vi "GUI AWG setup.vi"(11 "awg":T3={"AWG type"=enum."Agilent 331xxA to 332xxA", "FGEN Resource Name"="", "Source (Onboard Clock)"="OnboardClock", "FGEN Channel"="0", "awg lib session"={"type"=enum."Agilent 331xxA to 332xxA", "VISA"="", "enable 10MHz ref"=FALSE, "cmi ckd2"={"VISA"="", "clock source"=enum."Auto", "manual ref clk"=FALSE, "ref clock [Hz]"=0.0, "div mode"=enum."Set divisor directly"}, "cmi sync v3"={"VISA"="", "baud rate [bd/s]"=115200, "source"=enum."Auto", "hv range"=enum."1kV", "fsrc is fixed"=FALSE, "fsrc [Hz]"=10000000.0, "freq integ [s]"=1.0, "freq filter"=5, "trig level"=enum."TTL 5V", "chn1 mode"=enum."Source divider", "chn1 level"=enum."Positive 5V", "chn2 mode"=enum."Source divider", "chn2 level"=enum."Positive 5V", "chn2 div"=1, "chn3 mode"=enum."Chn 1 Active", "chn3 level"=enum."Positive 5V", "chn1 div entry"=enum."Calculate nearest divisor from measured fx", "chn1 dev limit [%]"=1.0, "chn1 check dev"=FALSE}, "trigger"={"source"=enum."Immediate", "level [V]"=0.0, "coupling"=enum."DC", "slope"=enum."POS"}, "HMF2500 cfg"={"Baud Rate"=9600, "Parity"=0, "Data Bits"=8, "Flow Control"=4}}} {"awg lib session"."HMF2500 cfg"."Flow Control" items=["None", "XON/XOFF", "RTS/CTS", "XON/XOFF & RTS/CTS", "DTR/DSR", "XON/XOFF & DTR/DSR"]; "awg lib session"."HMF2500 cfg"."Data Bits" items=["7"=7, "8"=8]; "awg lib session"."HMF2500 cfg"."Parity" items=["None", "Odd", "Even", "Mark", "Space"]; "awg lib session"."HMF2500 cfg"."Baud Rate" items=["300"=300, "600"=600, "1200"=1200, "2400"=2400, "4800"=4800, "9600"=9600, "19200"=19200]; "awg lib session"."cmi sync v3"."chn2 div" min=1 max=100000000 step=1; "awg lib session"."cmi sync v3"."fsrc [Hz]" format="%_8p"}) -> (3 "awg out":T3={"AWG type"=enum."Agilent 331xxA to 332xxA", "FGEN Resource Name"="", "Source (Onboard Clock)"="OnboardClock", "FGEN Channel"="0", "awg lib session"={"type"=enum."Agilent 331xxA to 332xxA", "VISA"="", "enable 10MHz ref"=FALSE, "cmi ckd2"={"VISA"="", "clock source"=enum."Auto", "manual ref clk"=FALSE, "ref clock [Hz]"=0.0, "div mode"=enum."Set divisor directly"}, "cmi sync v3"={"VISA"="", "baud rate [bd/s]"=115200, "source"=enum."Auto", "hv range"=enum."1kV", "fsrc is fixed"=FALSE, "fsrc [Hz]"=10000000.0, "freq integ [s]"=1.0, "freq filter"=5, "trig level"=enum."TTL 5V", "chn1 mode"=enum."Source divider", "chn1 level"=enum."Positive 5V", "chn2 mode"=enum."Source divider", "chn2 level"=enum."Positive 5V", "chn2 div"=1, "chn3 mode"=enum."Chn 1 Active", "chn3 level"=enum."Positive 5V", "chn1 div entry"=enum."Calculate nearest divisor from measured fx", "chn1 dev limit [%]"=1.0, "chn1 check dev"=FALSE}, "trigger"={"source"=enum."Immediate", "level [V]"=0.0, "coupling"=enum."DC", "slope"=enum."POS"}, "HMF2500 cfg"={"Baud Rate"=9600, "Parity"=0, "Data Bits"=8, "Flow Control"=4}}} {"awg lib session"."HMF2500 cfg"."Flow Control" items=["None", "XON/XOFF", "RTS/CTS", "XON/XOFF & RTS/CTS", "DTR/DSR", "XON/XOFF & DTR/DSR"]; "awg lib session"."HMF2500 cfg"."Data Bits" items=["7"=7, "8"=8]; "awg lib session"."HMF2500 cfg"."Parity" items=["None", "Odd", "Even", "Mark", "Space"]; "awg lib session"."HMF2500 cfg"."Baud Rate" items=["300"=300, "600"=600, "1200"=1200, "2400"=2400, "4800"=4800, "9600"=9600, "19200"=19200]; "awg lib session"."cmi sync v3"."chn2 div" min=1 max=100000000 step=1; "awg lib session"."cmi sync v3"."fsrc [Hz]" format="%_8p"})   [LabVIEW 2020]
doc: "Use this template to build a producer/consumer design pattern with events to produce queue items. Use this design pattern instead of the User Interface Event Handler pattern for user interfaces when you want to execute code asynchronously in response to an event without slowing the user interface responsiveness."
uses:
  General AWG/Type definitions/AWG.ctl
  General AWG/Type definitions/AWG type.ctl
  <instrlib>/niFgen/niFgen.llb/niFgen_ctl Sample Clock Source Values (Ring).ctl
  external libraries/AWG/AWG Session.ctl
  external libraries/AWG/AWG Type.ctl
  external libraries/AWG/CMI Clock Divider v2/CMI ckd2 Session.ctl
  external libraries/AWG/CMI Clock Divider v2/CMI ckd2 Source Mode.ctl
  external libraries/AWG/CMI Clock Divider v2/CMI ckd2 Divisor Mode.ctl
  external libraries/AWG/CMI Sync V3/CMI Sync V3 session.ctl
  external libraries/AWG/CMI Sync V3/Configure/CMI Sync V3 Reference Clock Source.ctl
  external libraries/AWG/CMI Sync V3/Configure/CMI Sync V3 HV input Range.ctl
  external libraries/AWG/CMI Sync V3/Configure/CMI Sync V3 Trigger Input Level.ctl
  external libraries/AWG/CMI Sync V3/Configure/CMI Sync V3 Channel 1 Mode.ctl
  external libraries/AWG/CMI Sync V3/Configure/CMI Sync V3 Channel Output Levels.ctl
  external libraries/AWG/CMI Sync V3/Configure/CMI Sync V3 Channel 2 Mode.ctl
  external libraries/AWG/CMI Sync V3/Configure/CMI Sync V3 Channel 3 Mode.ctl
  external libraries/AWG/CMI Sync V3/Configure/CMI Sync V3 Channel 1 Divisor Entry Mode.ctl
  external libraries/externals needed for AWG/ADC Trig Config.ctl
  external libraries/externals needed for AWG/ADC Trig Mode Source.ctl
  external libraries/externals needed for AWG/ADC Trig Coupling.ctl
  external libraries/externals needed for AWG/ADC Trig Slope.ctl
  external libraries/AWG/RaS HMF2500/HMF2500 Config.ctl
  <vilib>/Utility/error.llb/DialogType.ctl
  <vilib>/Utility/error.llb/Error Cluster From Error Code.vi
  <vilib>/ErrorRing/Error Ring.xnode
  external libraries/varilib/varilib.lvlib
  external libraries/AWG/AWG.lvlib
  external libraries/AWG/CMI Sync V3/CMI Sync Unit V3.lvlib
panel:
  in  "AWG type":T1
  in  "Channel":string
  in  "Clock Source":T2="OnboardClock"
  in  "FGEN Resource Name":refnum<k15>
  in  "Enable 10MHz ref":bool
  in  "VISA":refnum<visa-resource-name>
  in  "control panel":bool
  out "gui_elements":refnum<vi>[](array[refnum])
  out "Status":string
  in  "save_and_quit":bool
  in  "test":bool
  in  "cancel":bool
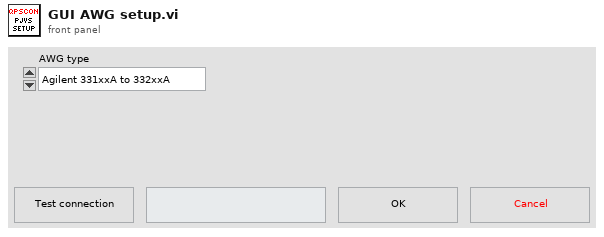
[diagram p1: front panel]
types:
  T1 = typedef "AWG type.ctl" = enum16{"Agilent 331xxA to 332xxA", "Agilent 335xxA to 336xxA", "Tektronix AFG3101C", "R&S HMF25xx", "CMI Clock Divider v2", "CMI Sync Unit V3", "FGEN NI 5413", "Supracon PJVS Generator", "dummy"}
  T2 = typedef "niFgen_ctl Sample Clock Source Values (Ring).ctl" = string
  T3 = typedef "AWG.ctl" = cluster{"AWG type":T1, "FGEN Resource Name":refnum<k15>, "Source (Onboard Clock)":T2, "FGEN Channel":string, "awg lib session":T4}
  T4 = typedef "AWG.lvlib/AWG Session.ctl" = cluster{"type":T5, "VISA":refnum<visa-resource-name>, "enable 10MHz ref":bool, "cmi ckd2":T6, "cmi sync v3":T9, "trigger":T18, "HMF2500 cfg":T22}
  T5 = typedef "AWG.lvlib/AWG Type.ctl" = enum16{"Agilent 331xxA to 332xxA", "Agilent 335xxA to 336xxA", "Tektronix AFG3101C", "R&S HMF25xx", "CMI Clock Divider v2", "CMI Sync Unit V3", "dummy"}
  T6 = typedef "AWG.lvlib/CMI ckd2 Session.ctl" = cluster{"VISA":refnum<visa-resource-name>, "clock source":T7, "manual ref clk":bool, "ref clock [Hz]":dbl, "div mode":T8}
  T7 = typedef "AWG.lvlib/CMI ckd2 Source Mode.ctl" = enum16{"Auto", "LF clock", "HF clock", "Internal"}
  T8 = typedef "AWG.lvlib/CMI ckd2 Divisor Mode.ctl" = enum16{"Set divisor directly", "Set divisor by frequency"}
  T9 = typedef "AWG.lvlib/CMI Sync Unit V3.lvlib/CMI Sync V3 session.ctl" = cluster{"VISA":refnum<visa-resource-name>, "baud rate [bd/s]":i32, "source":T10, "hv range":T11, "fsrc is fixed":bool, "fsrc [Hz]":dbl, "freq integ [s]":dbl, "freq filter":i32, "trig level":T12, "chn1 mode":T13, "chn1 level":T14, "chn2 mode":T15, "chn2 level":T14, "chn2 div":i32, "chn3 mode":T16, "chn3 level":T14, "chn1 div entry":T17, "chn1 dev limit [%]":dbl, "chn1 check dev":bool}
  T10 = typedef "AWG.lvlib/CMI Sync Unit V3.lvlib/CMI Sync V3 Reference Clock Source.ctl" = enum16{"Auto", "Internal", "Logic", "Sine", "HV"}
  T11 = typedef "AWG.lvlib/CMI Sync Unit V3.lvlib/CMI Sync V3 HV input Range.ctl" = enum16{"10V", "60V", "250V", "1kV"}
  T12 = typedef "AWG.lvlib/CMI Sync Unit V3.lvlib/CMI Sync V3 Trigger Input Level.ctl" = enum16{"LVCMOS 3V3", "TTL 5V"}
  T13 = typedef "AWG.lvlib/CMI Sync Unit V3.lvlib/CMI Sync V3 Channel 1 Mode.ctl" = enum16{"Source divider", "DDS absolute", "DDS ratio", "DDS ratio M/N"}
  T14 = typedef "AWG.lvlib/CMI Sync Unit V3.lvlib/CMI Sync V3 Channel Output Levels.ctl" = enum16{"Positive 3V3", "Negative 3V3", "Positive 5V", "Negative 5V"}
  T15 = typedef "AWG.lvlib/CMI Sync Unit V3.lvlib/CMI Sync V3 Channel 2 Mode.ctl" = enum16{"Source divider", "Chn 1 divide"}
  T16 = typedef "AWG.lvlib/CMI Sync Unit V3.lvlib/CMI Sync V3 Channel 3 Mode.ctl" = enum16{"Chn 1 Active", "Chn 2 Active", "Chn 1 Trigger", "Chn 2 Trigger", "Gate", "PPS", "10MHz"}
  T17 = typedef "AWG.lvlib/CMI Sync Unit V3.lvlib/CMI Sync V3 Channel 1 Divisor Entry Mode.ctl" = enum16{"Set divisor directly", "Calculate nearest divisor from measured fx"}
  T18 = typedef "ADC Trig Config.ctl" = cluster{"source":T19, "level [V]":dbl, "coupling":T20, "slope":T21}
  T19 = typedef "ADC Trig Mode Source.ctl" = enum16{"Immediate", "External", "Level"}
  T20 = typedef "ADC Trig Coupling.ctl" = enum16{"DC", "AC"}
  T21 = typedef "ADC Trig Slope.ctl" = enum16{"POS", "NEG"}
  T22 = typedef "AWG.lvlib/HMF2500 Config.ctl" = cluster{"Baud Rate":u32, "Parity":u16, "Data Bits":u16, "Flow Control":u16}
  T23 = typedef "DialogType.ctl" = u16
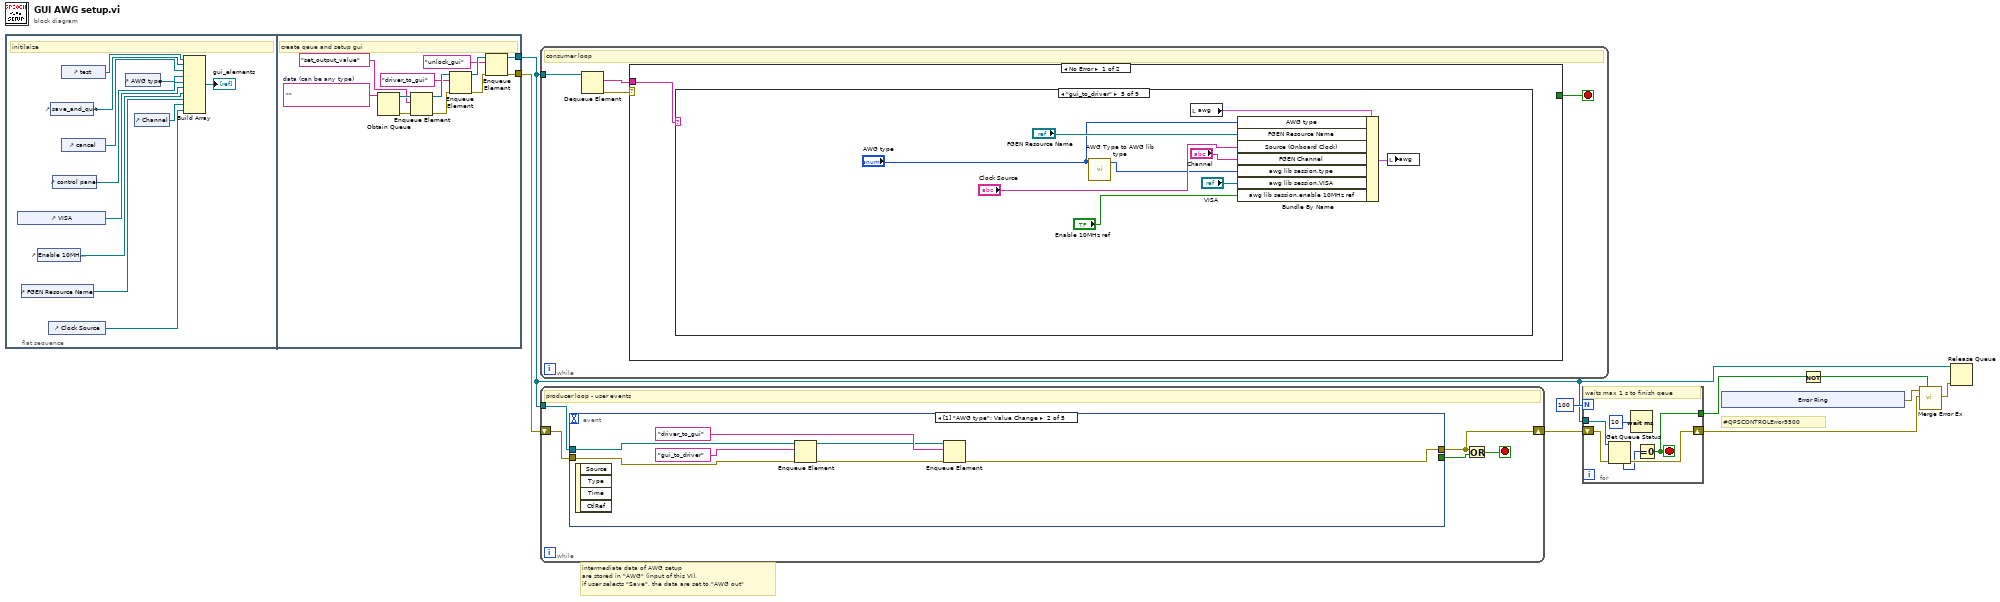
[diagram p0: block diagram]
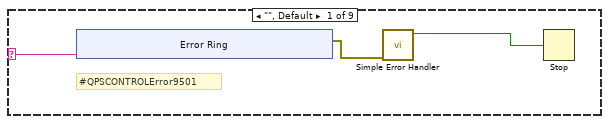
[diagram p2: hidden frame]
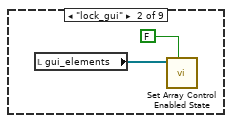
[diagram p3: hidden frame]
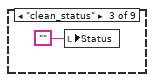
[diagram p4: hidden frame]
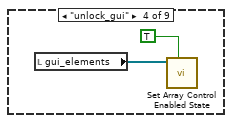
[diagram p5: hidden frame]
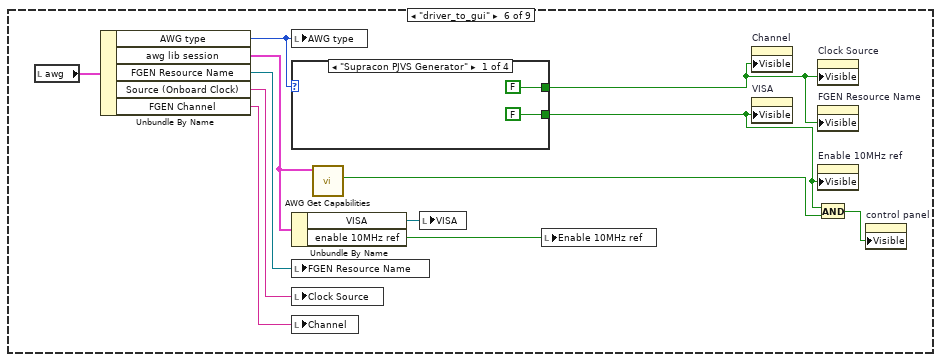
[diagram p6: hidden frame]
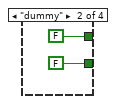
[diagram p7: hidden frame]
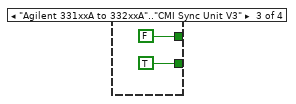
[diagram p8: hidden frame]
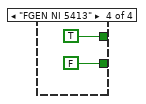
[diagram p9: hidden frame]
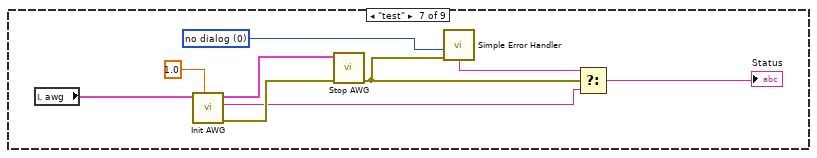
[diagram p10: hidden frame]
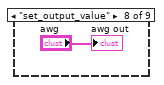
[diagram p11: hidden frame]
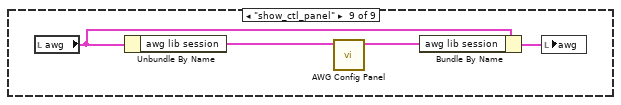
[diagram p12: hidden frame]
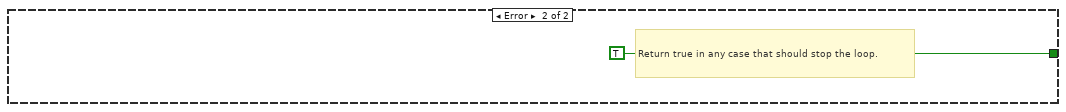
[diagram p13: hidden frame]
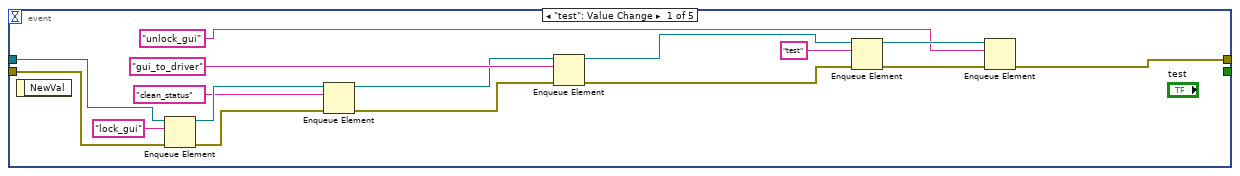
[diagram p14: hidden frame]
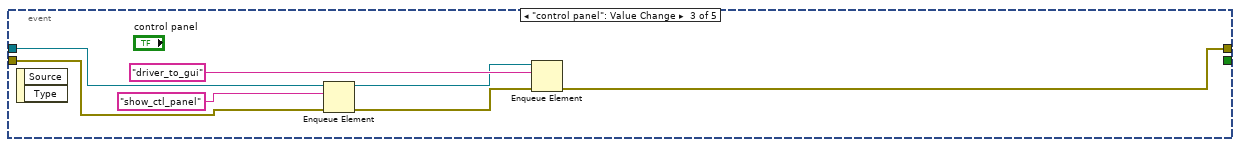
[diagram p15: hidden frame]
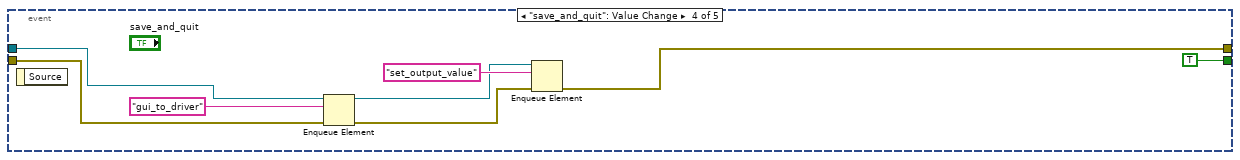
[diagram p16: hidden frame]
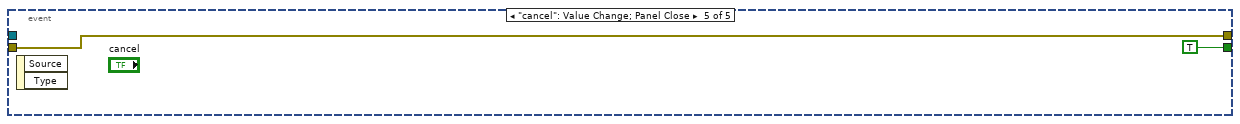
[diagram p17: hidden frame]
diagram:
  # "#QPSCONTROLError9500"
  # "intermediate data of AWG setup\nare stored in \"AWG\" (input of this VI),\nif user selects \"Save\", the data are set to \"AWG out\""
  n1 = flat-sequence {
    tunnel: [w23] -> w2
    tunnel: [w21] -> w1
    frame #0 {
      # "initilaize"
      n2 = control-ref of="VISA"() -> (w15:refnum<vi>)
      n3 = control-ref of="FGEN Resource Name"() -> (w13:refnum<vi>)
      n4 = control-ref of="Enable 10MHz ref"() -> (w14:refnum<vi>)
      n5 = control-ref of="Clock Source"() -> (w11:refnum<vi>)
      n6 = control-ref of="save_and_quit"() -> (w19:refnum<vi>)
      n7 = control-ref of="control panel"() -> (w16:refnum<vi>)
      n8 = control-ref of="test"() -> (w20:refnum<vi>)
      n9 = control-ref of="cancel"() -> (w18:refnum<vi>)
      n10 = control-ref of="AWG type"() -> (w10:refnum<vi>)
      n11 = control-ref of="Channel"() -> (w12:refnum<vi>)
      n12 = Build Array(w20, w19, w18, w10, w16, w15, w14, w13, w12, w11) -> (→"gui_elements":refnum<vi>[])
    }
    frame #1 {
      w22 = ""  # data (can be any type)
      # "create qeue and setup gui"
      n13 = Obtain Queue(element data type=w22) -> (queue out=w27:refnum<queue>, error out=w29:errorcluster)  [unwired: 4 in, 1 out]
      n14 = Enqueue Element(queue=w27, element="set_output_value", error in (no error)=w29) -> (queue out=w28:refnum<queue>, error out=w30:errorcluster)  [unwired: 1 in, 1 out]
      n15 = Enqueue Element(queue=w28, element="driver_to_gui", error in (no error)=w30) -> (queue out=w32:refnum<queue>, error out=w31:errorcluster)  [unwired: 1 in, 1 out]
      n16 = Enqueue Element(queue=w32, element="unlock_gui", error in (no error)=w31) -> (queue out=w23:refnum<queue>, error out=w21:errorcluster)  [unwired: 1 in, 1 out]
    }
  }
  n17 = while {
    tunnel: w2 -> [w36]
    stop <- w33 stop-if-true
    # "consumer loop"
    n18 = Dequeue Element(queue=w36) -> (element=w34:string, error out=w35:errorcluster)  [unwired: 2 in, 2 out]
    n19 = case shown="No Error" w35 {
      tunnel: w34 -> [w37 _]
      tunnel: [_ TRUE] -> w33
      frame No Error {
        n20 = case shown="\"gui_to_driver\"" w37 {
          selector: w37 -> [w38 _ _ _ _ _ _ _ _]
          frame "", Default {
            # "#QPSCONTROLError9501"
            n21 = xnode "Error Ring"("parameter 0"=w38) -> ("error out"=w40:errorcluster)
            n22 = call <vilib>:"Simple Error Handler.vi"("error in (no error)"=w40) -> ("error?"=w39:bool)  [unwired: 4 in, 4 out]
            n23 = Stop(stop? (T)=w39) -> ()
          }
          frame "lock_gui" {
            n24 = local read "gui_elements"() -> (w49:refnum<vi>[])
            n25 = call "Set Array Control Enabled State.vi"("enabled (T)"=FALSE, "reference array in"=w49) -> ()  [unwired: 8 in, 2 out]
          }
          frame "clean_status" {
            n26 = local write "Status"("") -> ()
          }
          frame "unlock_gui" {
            n27 = local read "gui_elements"() -> (w52:refnum<vi>[])
            n28 = call "Set Array Control Enabled State.vi"("enabled (T)"=TRUE, "reference array in"=w52) -> ()  [unwired: 8 in, 2 out]
          }
          frame "gui_to_driver" {
            n29 = call "AWG Type to AWG lib type.vi"("AWG type"="AWG type") -> ("AWG lib type"=w54:T5)  [unwired: 10 in]
            n30 = local read "awg"() -> (w60:T3)
            n31 = Bundle By Name(cluster=w60, "AWG type"="AWG type", "FGEN Resource Name"="FGEN Resource Name", "Source (Onboard Clock)"="Clock Source", "FGEN Channel"="Channel", "awg lib session.type"=w54, "awg lib session.VISA"="VISA", "awg lib session.enable 10MHz ref"="Enable 10MHz ref") -> (w61:T3)
            n32 = local write "awg"(w61) -> ()
          }
          frame "driver_to_gui" {
            n33 = local read "awg"() -> (w71:T3)
            n34 = Unbundle By Name(w71) -> ("AWG type"=w62:T1, "awg lib session"=w63:T4, "FGEN Resource Name"=w64:refnum<k15>, "Source (Onboard Clock)"=w65:T2, "FGEN Channel"=w66:string)
            n35 = local write "AWG type"(w62) -> ()
            n36 = case shown="\"Supracon PJVS Generator\"" w62 {
              tunnel: [FALSE ("x") FALSE ("x") TRUE ("x") FALSE ("x")] -> w68
              tunnel: [FALSE ("Visible") FALSE ("Visible") FALSE ("Visible") TRUE ("Visible")] -> w67
              frame "Supracon PJVS Generator" {
              }
              frame "dummy" {
              }
              frame "Agilent 331xxA to 332xxA".."CMI Sync Unit V3" {
              }
              frame "FGEN NI 5413" {
              }
            }
            n37 = Unbundle By Name(w63) -> ("VISA"=w72:refnum<visa-resource-name>, "enable 10MHz ref"=w73:bool)
            n38 = local write "FGEN Resource Name"(w64) -> ()
            n39 = local write "Clock Source"(w65) -> ()
            n40 = local write "Channel"(w66) -> ()
            n41 = call "AWG Get Capabilities.vi"("awg session"=w63) -> ("has cfg panel?"=w70:bool)  [unwired: 6 in, 4 out]
            n42 = local write "VISA"(w72) -> ()
            n43 = local write "Enable 10MHz ref"(w73) -> ()
            n44 = property on="Channel" class="Str"("Visible"=w67) -> ()  [unwired: 2 in, 2 out]
            n45 = property on="VISA" class="VISAName"("Visible"=w68) -> ()  [unwired: 2 in, 2 out]
            n46 = property on="Clock Source" class="CmbBox (strict)"("Visible"=w67) -> ()  [unwired: 2 in, 2 out]
            n47 = property on="FGEN Resource Name" class="IVIName"("Visible"=w67) -> ()  [unwired: 2 in, 2 out]
            n48 = property on="Enable 10MHz ref" class="Bool (strict)"("Visible"=w68) -> ()  [unwired: 2 in, 2 out]
            n49 = And(x=w68, y=w70) -> (x .and. y?=w69:bool)
            n50 = property on="control panel" class="Bool"("Visible"=w69) -> ()  [unwired: 2 in, 2 out]
          }
          frame "test" {
            w90 = T23 0 items=["no dialog", "OK message", "continue or stop message", "OK message + warnings", "continue/stop + warnings"] ("type of dialog (OK msg:1)")
            n51 = local read "awg"() -> (w87:T3)
            n52 = call "Init AWG.vi"("Trigger frequency  (Hz)"=1.0, "AWG"=w87) -> ("error out"=w84:errorcluster, "Init status"=w83:string, "AWG out"=w86:T3)  [unwired: 7 in]
            n53 = call "Stop AWG.vi"("error in (no error)"=w84, "AWG"=w86) -> ("error out"=w82:errorcluster)  [unwired: 8 in, 1 out]
            n54 = call <vilib>:"Simple Error Handler.vi"("type of dialog (OK msg:1)"=w90, "error in (no error)"=w82) -> ("message"=w89:string)  [unwired: 3 in, 4 out]
            n55 = Select(t=w89, s=w82, f=w83) -> (s? t:f=→"Status":string)
          }
          frame "set_output_value" {
            "awg out" <- "awg"
          }
          frame "show_ctl_panel" {
            n56 = local read "awg"() -> (w94:T3)
            n57 = Unbundle By Name(w94) -> ("awg lib session"=w95:T4)
            n58 = call "AWG Config Panel.vi"("awg session"=w95) -> ("awg session out"=w93:T4)  [unwired: 9 in, 1 out]
            n59 = Bundle By Name(cluster=w94, "awg lib session"=w93) -> (w92:T3)
            n60 = local write "awg"(w92) -> ()
          }
        }
      }
      frame Error {
        # "Return true in any case that should stop the loop."
      }
    }
  }
  n61 = while {
    shift-right: [w97] -> w5
    shift-left: w1 -> [w100]
    tunnel: w2 -> [w101]
    stop <- w98 stop-if-true
    # "producer loop - user events"
    n62 = event shown="[1] \"AWG type\": Value Change" {
      selector: _ -> [_ _ _ _ _]
      dyn-events: _ -> [_ _ _ _ _]
      timeout: _ -> [_ _ _ _ _]
      tunnel: w101 -> [w108 w123 w130 w136 _]
      tunnel: w100 -> [w109 w120 w127 w133 w141]
      tunnel: [w112 w118 w125 w132 w141] -> w97
      tunnel: [_ _ _ TRUE ("cancel") TRUE ("cancel")] -> w99
      event "test": Value Change {
        n63 = event-data() -> ()  [unwired: 1 in, 1 out]
        n64 = Enqueue Element(queue=w108, element="lock_gui", error in (no error)=w109) -> (queue out=w105:refnum<queue>, error out=w106:errorcluster)  [unwired: 1 in, 1 out]
        n65 = Enqueue Element(queue=w105, element="clean_status", error in (no error)=w106) -> (queue out=w103:refnum<queue>, error out=w104:errorcluster)  [unwired: 1 in, 1 out]
        n66 = Enqueue Element(queue=w103, element="gui_to_driver", error in (no error)=w104) -> (queue out=w115:refnum<queue>, error out=w116:errorcluster)  [unwired: 1 in, 1 out]
        n67 = Enqueue Element(queue=w115, element="test", error in (no error)=w116) -> (queue out=w111:refnum<queue>, error out=w113:errorcluster)  [unwired: 1 in, 1 out]
        n68 = Enqueue Element(queue=w111, element="unlock_gui", error in (no error)=w113) -> (error out=w112:errorcluster)  [unwired: 1 in, 2 out]
      }
      event Value Change {
        n69 = event-data() -> ()  [unwired: 1 in, 4 out]
        n70 = Enqueue Element(queue=w123, element="gui_to_driver", error in (no error)=w120) -> (queue out=w121:refnum<queue>, error out=w119:errorcluster)  [unwired: 1 in, 1 out]
        n71 = Enqueue Element(queue=w121, element="driver_to_gui", error in (no error)=w119) -> (error out=w118:errorcluster)  [unwired: 1 in, 2 out]
      }
      event "control panel": Value Change {
        n72 = event-data() -> ()  [unwired: 1 in, 2 out]
        n73 = Enqueue Element(queue=w130, element="show_ctl_panel", error in (no error)=w127) -> (queue out=w128:refnum<queue>, error out=w126:errorcluster)  [unwired: 1 in, 1 out]
        n74 = Enqueue Element(queue=w128, element="driver_to_gui", error in (no error)=w126) -> (error out=w125:errorcluster)  [unwired: 1 in, 2 out]
      }
      event "save_and_quit": Value Change {
        n75 = event-data() -> ()  [unwired: 1 in, 1 out]
        n76 = Enqueue Element(queue=w136, element="gui_to_driver", error in (no error)=w133) -> (queue out=w135:refnum<queue>, error out=w134:errorcluster)  [unwired: 1 in, 1 out]
        n77 = Enqueue Element(queue=w135, element="set_output_value", error in (no error)=w134) -> (error out=w132:errorcluster)  [unwired: 1 in, 2 out]
      }
      event "cancel": Value Change; Panel Close {
        n78 = event-data() -> ()  [unwired: 1 in, 2 out]
      }
    }
    n79 = Or(x=w97, y=w99) -> (x .or. y?=w98:bool)
  }
  n80 = for {
    N: 100 -> [_]
    tunnel: w2 -> [w147]
    shift-right: [w145] -> w6
    shift-left: w5 -> [w146]
    tunnel: [w142] -> w3
    stop <- w142 stop-if-true
    # "waits max 1 s to finish qeue"
    n81 = Get Queue Status(queue=w147, error in (no error)=w146) -> (error out=w145:errorcluster, # elements in queue=w143:i32)  [unwired: 1 in, 6 out]
    n82 = Wait (ms)(milliseconds to wait=u32 10) -> ()  [unwired: 1 out]
    n83 = Equal To 0?(x=w143) -> (x = 0?=w142:bool)
  }
  n84 = xnode "Error Ring"() -> ("error out"=w7:errorcluster)
  n85 = Not(x=w3) -> (.not. x?=w8:bool)
  n86 = call "Merge Error Ex.vi"("Is error? (False)"=w8, "main error in (no error)"=w6, "second error in"=w7) -> ("error out"=w4:errorcluster)  [unwired: 8 in]
  n87 = Release Queue(queue=w2, error in (no error)=w4) -> ()  [unwired: 1 in, 3 out]
